vi "DAQ NI USB-6211.vi"() -> ()   [LabVIEW 2011]
doc: "I. Description:\nThis example demonstrates how to continuously acquire data (Waveform) using the device's internal timing (rate is governed by an internally generated pulse train).\n\nII. Instructions for Running:\n1. Select the physical channel to correspond to where your signal is input on the DAQ device.\n2. Enter the minimum and maximum voltage ranges.\nNote: For better accuracy try to match the input range to the expected voltage level of the measured signal.\n3. Set the sample rate of the acquisition. Also set the Samples to Read control. This will determine how many samples are read each time the while loop iterates. This also determines how many points are plotted on the chart each iteration.\nNote: The rate should be at least twice as fast as the maximum frequency component of the signal being acquired.\n\n\nIII. Block Diagram Steps:\n1. Create an analog input voltage channel.\n2. Set the rate for the sample clock. Additionally, define the sample mode to be continuous.\n3. Call the Start VI to start acquiring samples.\n4. Read the waveform data in a loop until the user hits the stop\nbutton or an error occurs.\n5. Call the Clear Task VI to clear the Task.\n6. Use the popup dialog box to display an error if any.\n\nIV. I/O Connections Overview:\nMake sure your signal input terminal matches the Physical Channel I/O control."
uses:
  <vilib>/Utility/error.llb/DialogType.ctl
  <vilib>/DAQmx/read.llb/DAQmx Read (Analog 1D Wfm NChan NSamp).vi
  <vilib>/DAQmx/create/channels.llb/DAQmx Create Channel (AI-Voltage-Basic).vi
  <vilib>/DAQmx/configure/timing.llb/DAQmx Timing (Sample Clock).vi
  <vilib>/measure/madcrms.llb/Averaged DC-RMS for N Chan.vi
  <vilib>/DAQmx/miscellaneous.llb/DAQmx Fill In Error Info.vi
  <vilib>/Utility/file.llb/Write To Spreadsheet File (DBL).vi
  <vilib>/measure/NI_MAPro.lvlib
  <vilib>/Analysis/NI_AALBase.lvlib
  libs/AccCouchDB.dll
panel:
  out "DB_value":dbl
  in  "Stop 2":bool
  out "Abort 2":i32
  in  "CouchApp Title":string
  out "dt (s)":dbl=0.1 format="%.2f"
  in  "RSE mode":i32=10083
  in  "Units":i32=10065
  in  "Maximum Value":dbl=10.0 format="%0.2f"
  in  "Minimum Value":dbl=-10.0 format="%0.2f"
  in  "ADC Scale":tag="Voltage without offset"
  in  "Physical Channel":tag="Dev3/ai1" caption="Physical Channels"
  in  "Comments":string="DAC output connected to ADCinput"
  in  "New File":bool
  in  "File":path=path "self_offset"
  in  "Comment":string="test run"
  in  "File":path=path "C:/=Data=/test_stat.txt"
  out "Save Stat":bool
  in  "Stop":bool
  in  "Save Run":bool=TRUE
  in  "Config":bool=TRUE
  in  "Statistics":bool=TRUE
  in  "Data":bool=TRUE
  in  "Data File Folder":path=path "C:/=Data="
  in  "Clear Data":bool
  out "St. Dev.":dbl[](array[numeric])=[0.0606080295114447, 0.0, 0.0, 0.0606080295114447]
  in  "Points averaged":i16=100
  out "Mean (nT)":dbl[](array[numeric])=[-1.2274541861368804, 0.0, 0.0, 1.2274541861368804]
  out "All Data":dbl[][](graph)
  in  "Data points shown":i32=12000
  out "B0 (nT)":dbl[](graph)
  out "B1 (nT)":dbl[](graph)
  out "B2 (nT)":dbl[](graph)
  in  "Samples to Average":dbl=50.0 format="%0.0f"
  out "std B2 (nT)":dbl=-0.0 format="%#.2g"
  out "std B1 (nT)":dbl=-0.0 format="%#.2g"
  out "St. Dev. (nT)":dbl=0.47143069560419465 format="%#.2g"
  out "B2 (nT)":dbl format="%#.2g"
  in  "a2 calibration":dbl=7000.0 caption="calibration" format="%0.2f"
  in  "a2offset":dbl caption="offset" format="%2.2f"
  out "a2":waveform(dbl)(graph) caption="channel    0"
  out "B1 (nT)":dbl format="%#.2g"
  in  "a1 calibration":dbl=7000.0 caption="calibration" format="%0.2f"
  in  "a1offset":dbl caption="offset" format="%2.2f"
  out "a1":waveform(dbl)(graph) caption="channel    0"
  out "Value (nT)":dbl=-1.242184595069126 format="%#.2g"
  in  "a0 calibration":dbl=7000.0 caption="Scale" format="%0.2f"
  in  "a0 offset":dbl caption="Offset (nT)" format="%2.2f"
  in  "Samples":i32=5000
  in  "Rate":dbl=50000.0 caption="Sampling Rate" format="%0.2f"
  out "a0":waveform(dbl)(graph)={"t0"=timestamp(3442847991.7249203 s since 1904-01-01), "dt"=0.001, "Y"=[-0.6363965277538518, -1.2348193906035534, -1.0506892789527515, -0.7744941114925676, -1.0506892789617879, -0.8665591673052365, -0.8665591673150927, -0.7284615835763785, -1.0967218068681208, -0.8665591673118095, -1.0506892789593247, -0.9125916952230737, -0.8205266393997237, -1.372916974338166, -1.9253073092700397, -1.6951446697137253, -2.3396000604763247, -2.2015024767408953, -2.1554699488296345, -2.3396000604755014, -1.6491121418090244, -1.5110145580719536, -1.2348193906068397, -0.774494111490926, -0.9125916952263569, -0.5443314719337898, -1.1887868626890075, -1.3268844464236136, -0.6824290556667544, -1.418949502249427, -0.9586242231376179, -1.5570470859881393, -1.0046567510447773, -1.1427543347859548, -0.820526639399722, -0.7284615835771969, -0.8205266394005469, -1.0046567510488804, -1.0046567510423123, -1.2348193906027316, -0.9125916952263521, -1.1887868626914706, -1.5110145580694903, -1.418949502254352, -2.0634048930062843, -2.0634048930071107, -2.1554699488296345, -2.0634048930054676, -1.833242253451613, -1.464982030161511, -1.4649820301639742, -0.8205266393997253, -1.1427543347818483, -0.7744941114909244, -1.0046567510464188, -0.8665591673060598, -1.0506892789634295, -0.9586242231351529, -1.0506892789544013, -1.4189495022469603, -1.32688444642608, -1.188786862693114, -1.0967218068738704, -1.3268844464285434, -0.9586242231359747, -0.45226641610797985, -1.0506892789543965, -0.820526639398902, -1.188786862692289, -1.5110145580719536, -1.6030796138985852, -2.017372365095845, -2.017372365097487, -2.385632588383489, -2.3396000604738663, -2.0634048930062843, -1.833242253451613, -1.5110145580727736, -1.3268844464285434, -1.6030796138952987, -1.0506892789617863, -0.8665591673093429, -0.7744941114884611, -0.9586242231343297, -1.1427543347826699, -1.050689278960143, -0.7744941114901028, -0.7744941114884595, -1.096721806871407, -1.1427543347810298, -1.2808519185156357, -0.820526639399722, -0.9586242231343314, -0.5443314719272201, -1.3268844464244385, -0.5443314719296802, -0.6824290556675776, -1.4649820301590446, -1.464982030161511, -1.1427543347834899]} caption="channel    0"
  # "DAQ with ADS USB-4716"
  # "Data Aquisition Section"
  # "Input Channels Section"
  # "Data File"
  # "last"
  # "Statistics"
  # "B0"
  # "B0 (nT)"
  # "B1"
  # "B1 (nT)"
  # "B2 (nT)"
  # "B2"
  # "|B| (nT)"
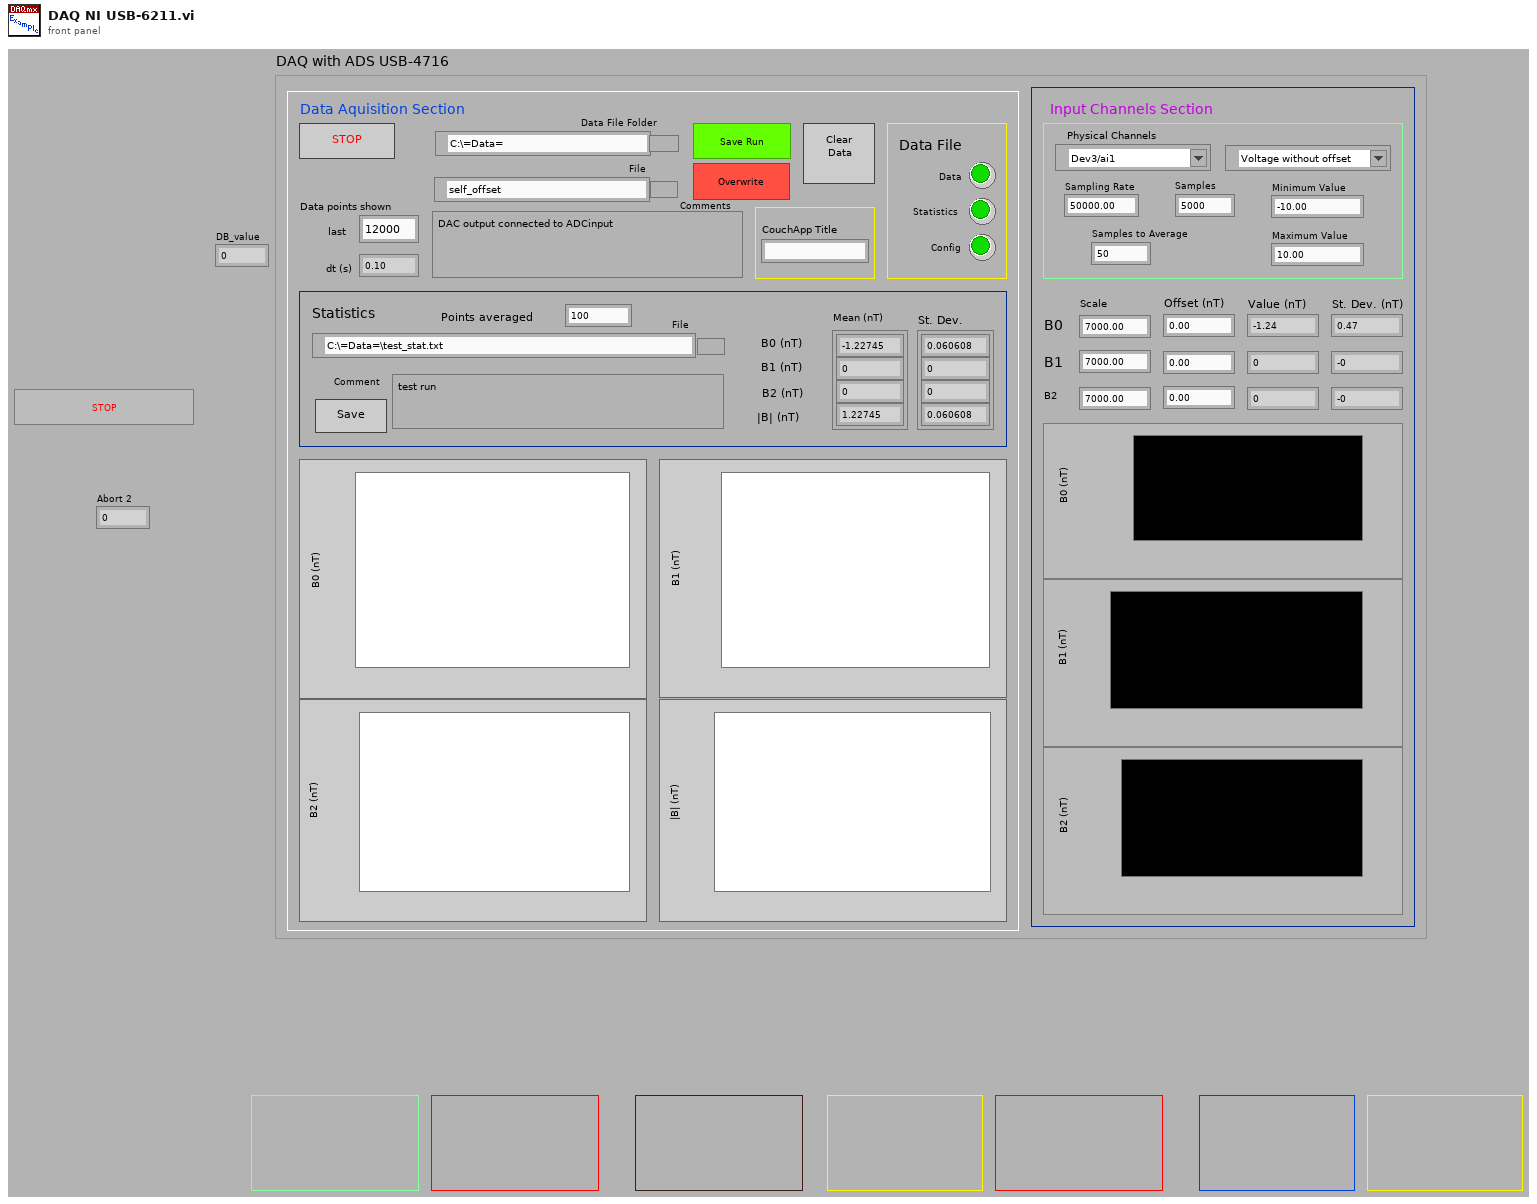
[diagram p1: front panel]
types:
  T1 = typedef "DialogType.ctl" = u16
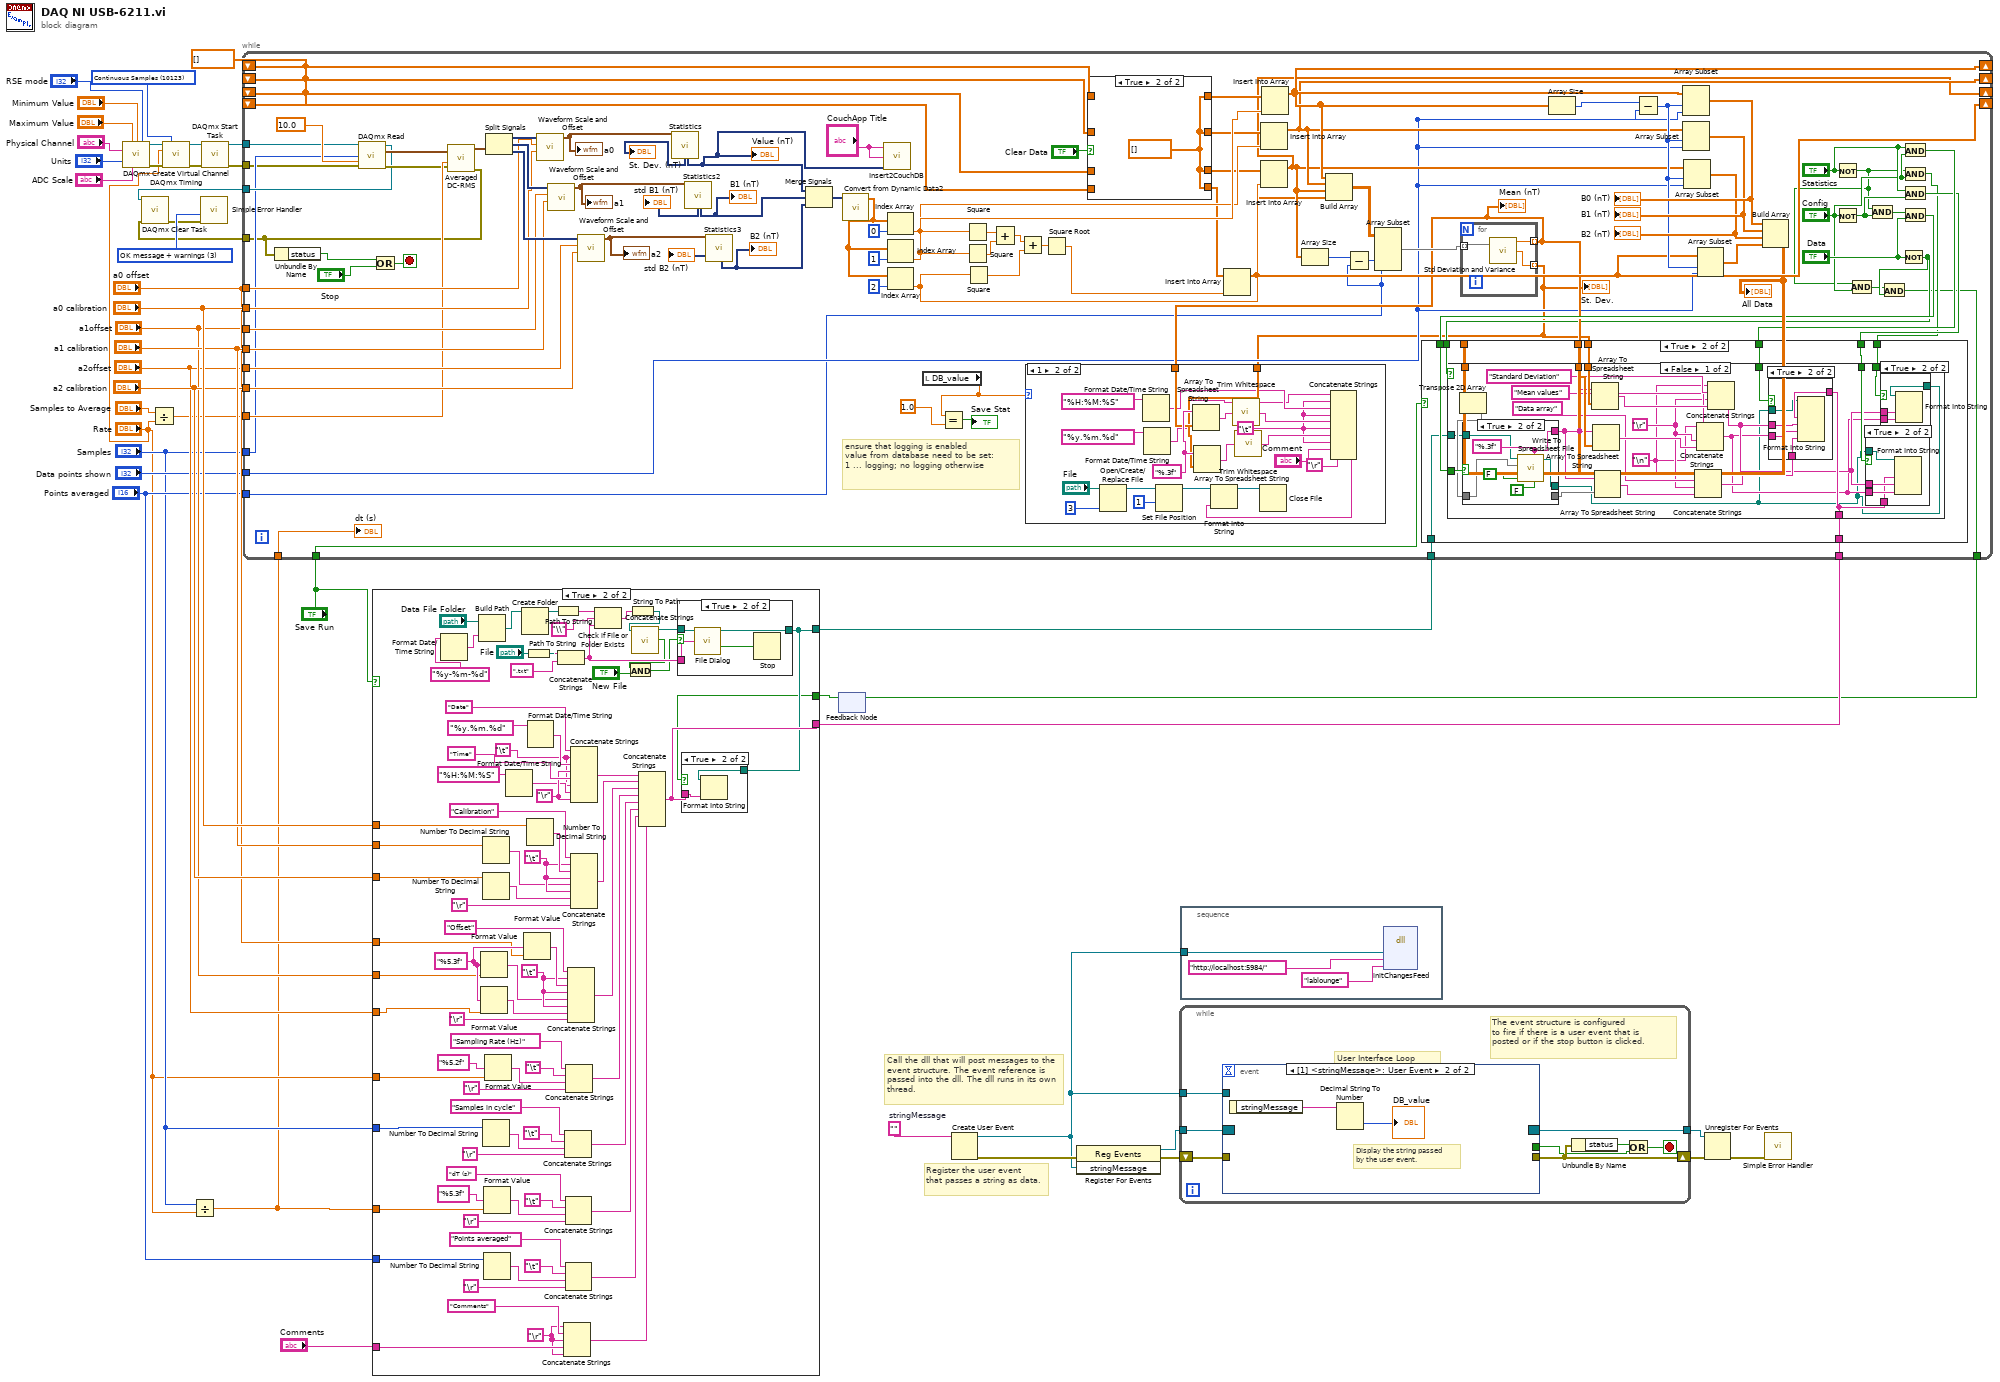
[diagram p0: block diagram]
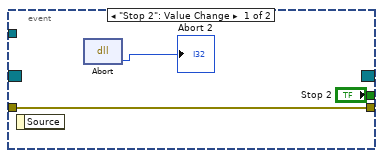
[diagram p2: hidden frame]
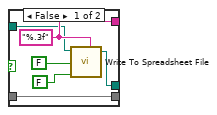
[diagram p8: hidden frame]
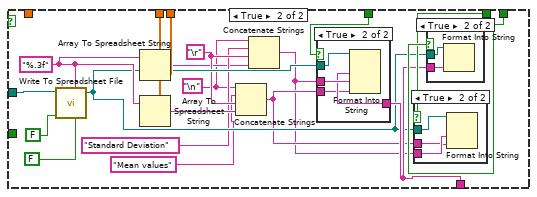
[diagram p12: hidden frame]
diagram:
  w2 = ""  # stringMessage
  w20 = 10123 items=["Finite Samples"=10178, "Continuous Samples"=10123] ("sample mode")
  w34 = T1 3 items=["no dialog", "OK message", "continue or stop message", "OK message + warnings", "continue/stop + warnings"] ("type of dialog (OK msg:1)")
  w37 = dbl[] []
  # "Call the dll that will post messages to the event structure. The event reference is passed into the dll. The dll runs in its own thread."
  # "Register the user event \nthat passes a string as data."
  n1 = call-poly <vilib>:"DAQmx Create Virtual Channel.vi"("maximum value"="Maximum Value", "minimum value"="Minimum Value", "input terminal configuration"="RSE mode", "physical channels"="Physical Channel", "units"="Units", "custom scale name"="ADC Scale") -> ("task out"=w22:refnum<k21>, "error out"=w21:errorcluster)  [unwired: 8 in]
  n2 = Divide(x="Samples to Average", y="Rate") -> (x/y=w39:dbl)
  n3 = call-poly <vilib>:"DAQmx Timing.vi"("task/channels in"=w22, "sample mode"=w20, "rate"="Rate", "error in"=w21) -> ("task out"=w19:refnum<k21>, "error out"=w18:errorcluster)  [unwired: 10 in]
  n4 = Divide(x="Samples", y="Rate") -> (x/y=w10:dbl)
  n5 = call <vilib>:"DAQmx Start Task.vi"("task/channels in"=w19, "error in"=w18) -> ("task out"=w24:refnum<k21>, "error out"=w23:errorcluster)  [unwired: 12 in]
  n6 = feedback #1() -> (w30:bool)  [unwired: 1 in]
  n7 = case shown="True" "Save Run" {
    tunnel: "a0 calibration" -> [_ w64]
    tunnel: "a1 calibration" -> [_ w65]
    tunnel: "a2 calibration" -> [_ w66]
    tunnel: "a0 offset" -> [_ w51]
    tunnel: "a1offset" -> [_ w50]
    tunnel: "a2offset" -> [_ w53]
    tunnel: "Samples" -> [_ w67]
    tunnel: "Rate" -> [_ w54]
    tunnel: w10 -> [_ w63]
    tunnel: "Points averaged" -> [_ w68]
    tunnel: [_ w57] -> w33
    tunnel: [_ w58] -> w32
    tunnel: w30 -> [_ w56]
    tunnel: "Comments" -> [_ w48]
    frame False {
    }
    frame True {
      w46 = "\r"
      w52 = "%5.3f"
      w92 = "\t"
      w100 = "\t"
      w106 = "\r"
      w104 = "\t"
      n8 = Format Date/Time String(time format string (%c)="%y-%m-%d") -> (date/time string=w120:string)  [unwired: 2 in]
      n9 = Build Path(base path="Data File Folder", name or relative path=w120) -> (appended path=w117:path)
      n10 = Format Value(format string=w52, value (0)=w50) -> (output string=w91:string)  [unwired: 1 in]
      n11 = Format Value(format string=w52, value (0)=w53) -> (output string=w90:string)  [unwired: 1 in]
      n12 = Number To Decimal String(number=w65) -> (decimal integer string=w99:string)  [unwired: 1 in]
      n13 = Number To Decimal String(number=w66) -> (decimal integer string=w98:string)  [unwired: 1 in]
      n14 = Number To Decimal String(number=w67) -> (decimal integer string=w84:string)  [unwired: 1 in]
      n15 = Format Value(format string="%5.3f", value (0)=w63) -> (output string=w78:string)  [unwired: 1 in]
      n16 = Number To Decimal String(number=w68) -> (decimal integer string=w74:string)  [unwired: 1 in]
      n17 = Format Value(format string="%5.2f", value (0)=w54) -> (output string=w88:string)  [unwired: 1 in]
      n18 = Format Date/Time String(time format string (%c)="%H:%M:%S") -> (date/time string=w105:string)  [unwired: 2 in]
      n19 = Create Folder(path (use dialog)=w117) -> (created path=w116:path)  [unwired: 2 in, 2 out]
      n20 = Format Value(format string=w52, value (0)=w51) -> (output string=w93:string)  [unwired: 1 in]
      n21 = Path To String(path="File") -> (string=w115:string)
      n22 = Number To Decimal String(number=w64) -> (decimal integer string=w101:string)  [unwired: 1 in]
      n23 = Format Date/Time String(time format string (%c)="%y.%m.%d") -> (date/time string=w109:string)  [unwired: 2 in]
      n24 = Path To String(path=w116) -> (string=w119:string)
      n25 = Concatenate Strings(w115, ".txt" ("string")) -> (w113:string)
      n26 = Concatenate Strings(w46, "Comments", w46, w48, w46) -> (w47:string)
      n27 = Concatenate Strings("Samples in cycle", "\t", w84, "\r") -> (w79:string)
      n28 = Concatenate Strings("dT (s)", "\t", w78, "\r") -> (w70:string)
      n29 = Concatenate Strings("Points averaged", "\t", w74, "\r") -> (w69:string)
      n30 = Concatenate Strings("Sampling Rate (Hz)", "\t", w88, "\r") -> (w80:string)
      n31 = Concatenate Strings("Offset", w92, w93, w92, w91, w92, w90, "\r") -> (w89:string)
      n32 = Concatenate Strings("Date", w104, w109, w106, "Time", w104, w105, w106) -> (w97:string)
      n33 = Concatenate Strings("Calibration", w100, w101, w100, w99, w100, w98, "\r") -> (w96:string)
      n34 = Concatenate Strings(w119, "\\" ("string"), w113) -> (w122:string)
      n35 = String To Path(string=w122) -> (path=w124:path)
      n36 = call <vilib>:"Check if File or Folder Exists.vi"("path"=w124) -> ("file or folder exists?"=w61:bool, "dup path"=w60:path)  [unwired: 8 in, 1 out]
      n37 = And(x=w61, y="New File") -> (x .and. y?=w59:bool)
      n38 = Concatenate Strings(w97, w96, w89, w80, w79, w70, w69, w47) -> (w58:string)
      n39 = case shown="True" w59 {
        tunnel: w113 -> [_ w132]
        tunnel: w60 -> [w128 w131]
        tunnel: [w128 w130] -> w57
        frame False {
        }
        frame True {
          n40 = call "File Dialog"("start path"=w131, "default name"=w132) -> ("selected path"=w130:path, "cancelled"=w129:bool)  [unwired: 10 in, 2 out]
          n41 = Stop(stop? (T)=w129) -> ()
        }
      }
      n42 = case shown="True" w56 {
        tunnel: w58 -> [_ w127]
        tunnel: w57 -> [_ w126]
        frame False {
        }
        frame True {
          n43 = Format Into String(initial string=w126, w127) -> ()  [unwired: 2 in, 2 out]
        }
      }
    }
  }
  n44 = while {
    tunnel: "Samples" -> [w142]
    tunnel: "a0 offset" -> [w223]
    tunnel: "a0 calibration" -> [w222]
    tunnel: "a1offset" -> [w221]
    tunnel: "a1 calibration" -> [w220]
    tunnel: "a2offset" -> [w219]
    tunnel: "a2 calibration" -> [w218]
    tunnel: w39 -> [w213]
    shift-right: [w180] -> _
    shift-left: w37 -> [w184]
    shift-right: [w179] -> _
    shift-left: w37 -> [w183]
    shift-right: [w172] -> _
    shift-left: w37 -> [w182]
    shift-right: [w171] -> _
    shift-left: w37 -> [w181]
    tunnel: "Points averaged" -> [w149]
    tunnel: "Data points shown" -> [w150]
    tunnel: "Save Run" -> [w168]
    tunnel: [w139] -> w26
    tunnel: w32 -> [w158]
    tunnel: w33 -> [w156]
    tunnel: [w151] -> w31
    tunnel: [w145] -> w25
    tunnel: w24 -> [w141]
    tunnel: w23 -> [w140]
    tunnel: w10 -> [w138]
    stop <- w157 stop-if-true
    # "ensure that logging is enabled\nvalue from database need to be set: \n1 ... logging; no logging otherwise"
    n45 = call-poly <vilib>:"DAQmx Read.vi"("task/channels in"=w141, "number of samples per channel"=w142, "timeout"=10.0 ("timeout (s)"), "error in"=w140) -> ("task out"=w145:refnum<k21>, "data"=w147:waveform(dbl)[], "error out"=w146:errorcluster)  [unwired: 9 in]
    n46 = call-poly <vilib>:"Averaged DC-RMS.vi"("error in (no error)"=w146, "averaging time"=w213, "signals in"=w147) -> ("error out"=w139:errorcluster, "DC value waveforms"=w214:waveform(dbl)[])  [unwired: 4 in, 3 out]
    n47 = Unbundle By Name(w139) -> ("status"=w169:bool)
    n48 = Or(x=w169, y="Stop") -> (x .or. y?=w157:bool)
    n49 = Split Signals(w214) -> (w226:dynamicdata, w224:dynamicdata, w225:dynamicdata)  [unwired: 3 in]
    n50 = call <vilib>:"Waveform Scale and Offset.vi"("scale"=w222, "offset"=w223, "waveform in"=w226) -> ("waveform out"=w176:waveform(dbl))  [unwired: 7 in, 1 out]
    "a0" <- w176
    n51 = call <vilib>:"Waveform Scale and Offset.vi"("scale"=w220, "offset"=w221, "waveform in"=w224) -> ("waveform out"=w175:waveform(dbl))  [unwired: 7 in, 1 out]
    "a1" <- w175
    n52 = call <vilib>:"Waveform Scale and Offset.vi"("scale"=w218, "offset"=w219, "waveform in"=w225) -> ("waveform out"=w174:waveform(dbl))  [unwired: 7 in, 1 out]
    "a2" <- w174
    n53 = call "Statistics"("Signals"=w176) -> ("Standard Dev"=→"St. Dev. (nT)":dynamicdata, "Arithmetic Mean"=w137:dynamicdata)  [unwired: 23 in, 2 out]
    "Value (nT)" <- w137
    n54 = call "Statistics2"("Signals"=w175) -> ("Standard Dev"=→"std B1 (nT)":dynamicdata, "Arithmetic Mean"=w212:dynamicdata)  [unwired: 24 in, 1 out]
    "B1 (nT)" <- w212
    n55 = call "Statistics3"("Signals"=w174) -> ("Standard Dev"=→"std B2 (nT)":dynamicdata, "Arithmetic Mean"=w211:dynamicdata)  [unwired: 24 in, 1 out]
    "B2 (nT)" <- w211
    n56 = Merge Signals(w137, w212, w211) -> (w177:dynamicdata)
    n57 = call "Convert from Dynamic Data2"("Dynamic Data Type"=w177) -> ("Array"=w173:dbl[])  [unwired: 3 in]
    n58 = call "Insert2CouchDB.vi"("value"=w137, "title"="CouchApp Title", "name"="CouchApp Title") -> ()
    n59 = Index Array(array=w173, index=0) -> (element=w197:dbl)
    n60 = Index Array(array=w173, index=1) -> (element=w196:dbl)
    n61 = Index Array(array=w173, index=2) -> (element=w195:dbl)
    n62 = local read "DB_value"() -> (w134:dbl)
    n63 = Equal?(x=w134, y=1.0) -> (x = y?=→"Save Stat":bool)
    n64 = Square(x=w197) -> (x^2=w203:dbl)
    n65 = Square(x=w196) -> (x^2=w202:dbl)
    n66 = Square(x=w195) -> (x^2=w199:dbl)
    n67 = Add(x=w203, y=w202) -> (x+y=w200:dbl)
    n68 = Add(x=w200, y=w199) -> (x+y=w201:dbl)
    n69 = Square Root(x=w201) -> (sqrt(x)=w198:dbl)
    n70 = case shown="True" "Clear Data" {
      tunnel: w184 -> [w337 _]
      tunnel: [w337 w338] -> w187
      tunnel: [w336 w338] -> w186
      tunnel: [w335 w338] -> w185
      tunnel: [w334 w338] -> w178
      tunnel: w183 -> [w336 _]
      tunnel: w182 -> [w335 _]
      tunnel: w181 -> [w334 _]
      frame False {
      }
      frame True {
        w338 = dbl[] []
      }
    }
    n71 = Insert Into Array(array=w178, new element=w198) -> (w171:dbl[])  [unwired: 1 in]
    n72 = Insert Into Array(array=w186, new element=w196) -> (w179:dbl[])  [unwired: 1 in]
    n73 = Insert Into Array(array=w185, new element=w195) -> (w172:dbl[])  [unwired: 1 in]
    n74 = Insert Into Array(array=w187, new element=w197) -> (w180:dbl[])  [unwired: 1 in]
    n75 = Array Size(array=w172) -> (size(s)=w190:i32)
    n76 = Build Array(w180, w179, w172, w171) -> (w192:dbl[][])
    n77 = Subtract(x=w190, y=w149) -> (x-y=w189:i32)
    n78 = Array Subset(array=w192, index (col)=w189, length (col)=w149) -> (w191:dbl[][])  [unwired: 2 in]
    n79 = for {
      tunnel: w191 -> [w340] mode=indexing
      tunnel: [w341] -> w159 mode=indexing
      tunnel: [w339] -> w148 mode=indexing
      n80 = call <vilib>:"Std Deviation and Variance.vi"("X"=w340) -> ("mean"=w341:dbl, "standard deviation"=w339:dbl)  [unwired: 1 in, 1 out]
    }
    "Mean (nT)" <- w159
    "St. Dev." <- w148
    n81 = case shown="1" w134 {
      tunnel: w159 -> [_ w241]
      tunnel: w148 -> [_ w240]
      frame 0, Default {
      }
      frame 1 {
        w229 = "\t"
        w242 = "%.3f" ("format (%.3f)")
        n82 = Open/Create/Replace File(file path (use dialog)="File", operation (0:open)=3) -> (refnum out=w245:refnum<file>)  [unwired: 4 in, 2 out]
        n83 = Format Date/Time String(time format string (%c)="%H:%M:%S") -> (date/time string=w233:string)  [unwired: 2 in]
        n84 = Format Date/Time String(time format string (%c)="%y.%m.%d") -> (date/time string=w227:string)  [unwired: 2 in]
        n85 = Set File Position(refnum=w245, from (0:start)=1) -> (refnum out=w244:refnum<file>)  [unwired: 2 in, 1 out]
        n86 = Array To Spreadsheet String(array=w241, 3:w242) -> (spreadsheet string=w235:string)  [unwired: 1 in]
        n87 = Array To Spreadsheet String(array=w240, 3:w242) -> (spreadsheet string=w236:string)  [unwired: 1 in]
        n88 = call <vilib>:"Trim Whitespace.vi"("string"=w235) -> ("trimmed string"=w232:string)  [unwired: 1 in]
        n89 = call <vilib>:"Trim Whitespace.vi"("string"=w236) -> ("trimmed string"=w231:string)  [unwired: 1 in]
        n90 = Concatenate Strings(w227, w229, w233, w229, w232, w229, w231, w229, "Comment", "\r") -> (w247:string)
        n91 = Format Into String(initial string=w244, w247) -> (resulting string=w243:refnum<file>)  [unwired: 2 in, 1 out]
        n92 = Close File(refnum=w243) -> ()  [unwired: 1 in, 2 out]
      }
    }
    n93 = Array Size(array=w180) -> (size(s)=w210:i32)
    n94 = Subtract(x=w210, y=w150) -> (x-y=w194:i32)
    n95 = Array Subset(array=w180, index=w194, length=w150) -> (w209:dbl[])
    "B0 (nT)" <- w209
    n96 = Array Subset(array=w179, index=w194, length=w150) -> (w208:dbl[])
    "B1 (nT)" <- w208
    n97 = Array Subset(array=w172, index=w194, length=w150) -> (w207:dbl[])
    "B2 (nT)" <- w207
    n98 = Array Subset(array=w171, index=w194, length=w150) -> (w193:dbl[])
    n99 = Build Array(w209, w208, w207, w193) -> (w170:dbl[][])
    "All Data" <- w170
    n100 = Not(x="Statistics") -> (.not. x?=w152:bool)
    n101 = Not(x="Config") -> (.not. x?=w163:bool)
    n102 = And(x=w152, y="Config") -> (x .and. y?=w154:bool)
    n103 = And(x=w152, y=w163) -> (x .and. y?=w167:bool)
    n104 = Not(x="Data") -> (.not. x?=w155:bool)
    n105 = And(x=w154, y=w155) -> (x .and. y?=w151:bool)
    n106 = And(x="Statistics", y="Config") -> (x .and. y?=w165:bool)
    n107 = And(x=w152, y="Config") -> (x .and. y?=w161:bool)
    n108 = And(x="Statistics", y=w163) -> (x .and. y?=w162:bool)
    n109 = And(x=w167, y="Data") -> (x .and. y?=w160:bool)
    n110 = case shown="True" w168 {
      tunnel: w148 -> [_ w257]
      tunnel: w159 -> [_ w256]
      tunnel: w155 -> [_ w255]
      tunnel: w170 -> [_ w254]
      tunnel: w165 -> [_ w253]
      tunnel: w162 -> [_ w252]
      tunnel: w161 -> [_ w251]
      tunnel: w160 -> [_ w250]
      tunnel: w158 -> [_ w249]
      tunnel: w156 -> [_ w248]
      frame False {
      }
      frame True {
        n111 = case shown="False" w255 {
          tunnel: w257 -> [w281 w323]
          tunnel: w256 -> [w280 w322]
          tunnel: w254 -> [w266 _]
          tunnel: w253 -> [w279 w319]
          tunnel: w252 -> [w278 w317]
          tunnel: w251 -> [w277 w318]
          tunnel: w250 -> [w276 _]
          tunnel: w249 -> [w262 w316]
          tunnel: w248 -> [w259 w314]
          frame False {
            w268 = "\r"
            w267 = "\n"
            n112 = Transpose 2D Array(2D array=w266) -> (transposed array=w265:dbl[][])
            n113 = case shown="True" w276 {
              tunnel: w265 -> [w287 w291]
              tunnel: [w287 _] -> w264
              tunnel: [w284 w290] -> w263
              tunnel: w259 -> [w282 w289]
              tunnel: [w283 w288] -> w258
              frame False {
                w284 = "%.3f" ("format (%.3f)")
                n114 = call-poly <vilib>:"Write To Spreadsheet File.vi"("transpose? (no:F)"=FALSE ("append to file? (new file:F)"), "format (%.3f)"=w284, "append to file? (new file:F)"=FALSE, "file path (dialog if empty)"=w282) -> ("new file path (Not A Path if cancelled)"=w283:path)  [unwired: 4 in]
              }
              frame True {
                w290 = "%.3f" ("format (%.3f)")
                n115 = call-poly <vilib>:"Write To Spreadsheet File.vi"("transpose? (no:F)"=FALSE ("append to file? (new file:F)"), "format (%.3f)"=w290, "append to file? (new file:F)"=FALSE, "2D data"=w291, "file path (dialog if empty)"=w289) -> ("new file path (Not A Path if cancelled)"=w288:path)  [unwired: 3 in]
              }
            }
            n116 = Array To Spreadsheet String(array=w281, 3:w263) -> (spreadsheet string=w272:string)  [unwired: 1 in]
            n117 = Array To Spreadsheet String(array=w280, 3:w263) -> (spreadsheet string=w274:string)  [unwired: 1 in]
            n118 = Array To Spreadsheet String(array=w264, 3:w263) -> (spreadsheet string=w269:string)  [unwired: 1 in]
            n119 = Concatenate Strings(w267, "Data array", w268, w269) -> (w275:string)
            n120 = Concatenate Strings(w267, "Mean values", w268, w274) -> (w260:string)
            n121 = Concatenate Strings(w267, "Standard Deviation", w268, w272) -> (w261:string)
            n122 = case shown="True" w279 {
              tunnel: w261 -> [_ w298]
              tunnel: w260 -> [_ w297]
              tunnel: w275 -> [_ w296]
              tunnel: w262 -> [_ w295]
              tunnel: w258 -> [_ w294]
              frame False {
              }
              frame True {
                n123 = Format Into String(initial string=w294, w295, w298, w297, w296) -> ()  [unwired: 2 in, 2 out]
              }
            }
            n124 = case shown="True" w278 {
              tunnel: w261 -> [_ w305]
              tunnel: w260 -> [_ w304]
              tunnel: w262 -> [_ w303]
              tunnel: w258 -> [_ w302]
              frame False {
              }
              frame True {
                n125 = Format Into String(initial string=w302, w303, w305, w304) -> ()  [unwired: 2 in, 2 out]
              }
            }
            n126 = case shown="True" w277 {
              tunnel: w261 -> [_ w301]
              tunnel: w260 -> [_ w300]
              tunnel: w258 -> [_ w299]
              frame False {
              }
              frame True {
                n127 = Format Into String(initial string=w299, w301, w300) -> ()  [unwired: 2 in, 2 out]
              }
            }
          }
          frame True {
            w306 = "\n"
            w313 = "\r"
            w320 = "%.3f" ("format (%.3f)")
            n128 = call-poly <vilib>:"Write To Spreadsheet File.vi"("transpose? (no:F)"=FALSE ("append to file? (new file:F)"), "format (%.3f)"=w320, "append to file? (new file:F)"=FALSE, "file path (dialog if empty)"=w314) -> ("new file path (Not A Path if cancelled)"=w315:path)  [unwired: 4 in]
            n129 = Array To Spreadsheet String(array=w323, 3:w320) -> (spreadsheet string=w307:string)  [unwired: 1 in]
            n130 = Array To Spreadsheet String(array=w322, 3:w320) -> (spreadsheet string=w311:string)  [unwired: 1 in]
            n131 = Concatenate Strings(w306, "Mean values", w313, w311) -> (w312:string)
            n132 = Concatenate Strings(w306, "Standard Deviation", w313, w307) -> (w308:string)
            n133 = case shown="True" w319 {
              tunnel: w308 -> [_ w328]
              tunnel: w315 -> [_ w327]
              tunnel: w316 -> [_ w326]
              tunnel: w312 -> [_ w325]
              frame False {
              }
              frame True {
                n134 = Format Into String(initial string=w327, w326, w328, w325) -> ()  [unwired: 2 in, 2 out]
              }
            }
            n135 = case shown="True" w317 {
              tunnel: w308 -> [_ w333]
              tunnel: w315 -> [_ w332]
              tunnel: w312 -> [_ w331]
              frame False {
              }
              frame True {
                n136 = Format Into String(initial string=w332, w333, w331) -> ()  [unwired: 2 in, 2 out]
              }
            }
            n137 = case shown="True" w318 {
              tunnel: w315 -> [_ w330]
              tunnel: w316 -> [_ w329]
              frame False {
              }
              frame True {
                n138 = Format Into String(initial string=w330, w329) -> ()  [unwired: 2 in, 2 out]
              }
            }
          }
        }
      }
    }
    "dt (s)" <- w138
  }
  n139 = call <vilib>:"DAQmx Clear Task.vi"("task in"=w25, "error in"=w26) -> ("error out"=w27:errorcluster)  [unwired: 13 in]
  n140 = call <vilib>:"Simple Error Handler.vi"("type of dialog (OK msg:1)"=w34, "error in (no error)"=w27) -> ()  [unwired: 3 in, 5 out]
  n141 = feedback-in #1(w31) -> ()
  n142 = Create User Event(user event datatype=w2) -> (user event=w3:refnum<user-event>, error out=w4:errorcluster)  [unwired: 1 in]
  n143 = register-events(error in=w4, w3) -> (reference out=w7:refnum<event-registration>, error out=w5:errorcluster)  [unwired: 1 in]
  n144 = while {
    tunnel: w7 -> [w349]
    shift-right: [w347] -> w8
    shift-left: w5 -> [w348]
    tunnel: [w346] -> w6
    tunnel: w3 -> [w342]
    stop <- w344 stop-if-true
    # "The event structure is configured\nto fire if there is a user event that is\nposted or if the stop button is clicked."
    # "User Interface Loop"
    n145 = event shown="[1] <stringMessage>: User Event" {
      selector: w349 -> [_ _]
      dyn-events: [_ _] -> w346
      timeout: _ -> [_ _]
      tunnel: ["Stop 2" _] -> w343
      tunnel: w348 -> [w351 _]
      tunnel: [w351 _] -> w347
      tunnel: w342 -> [_ _]
      event "Stop 2": Value Change {
        n146 = event-data() -> ()  [unwired: 1 in, 1 out]
        n147 = dll-call lib="C:/projects/libs/AccCouchDB.dll" fn="Abort"() -> ("return type"=→"Abort 2":i32)  [unwired: 3 in, 2 out]
      }
      event User Event {
        # "Display the string passed\nby the user event."
        n148 = event-data() -> ("stringMessage"=w354:string)  [unwired: 1 in]
        n149 = Decimal String To Number(string=w354) -> (number=→"DB_value":i32)  [unwired: 2 in, 1 out]
      }
    }
    n150 = Unbundle By Name(w347) -> ("status"=w345:bool)
    n151 = Or(x=w345, y=w343) -> (x .or. y?=w344:bool)
  }
  n152 = stacked-sequence {
    tunnel: w3 -> [w357]
    frame #0 {
      n153 = dll-call lib="C:/projects/libs/AccCouchDB.dll" fn="initChangesFeed"("UserEventRef"=w357, "server"="http://localhost:5984/", "database"="lablounge") -> ()  [unwired: 7 in, 2 out]
    }
  }
  n154 = Unregister For Events(event registration refnum=w6, error in=w8) -> (error out=w9:errorcluster)
  n155 = call <vilib>:"Simple Error Handler.vi"("error in (no error)"=w9) -> ()  [unwired: 4 in, 5 out]
